vi "CAL-Get MAX SPL (tone, scalar).vi"(0 "Cal Path":path, 7 "Frequency (kHz)":dbl, 11 "error in (no error)":errorcluster) -> (8 "Max SPL":dbl, 15 "error out":errorcluster)   [LabVIEW 2020]
uses:
  PXI DAQ VIs/DAQ Engine VIs/PXI Globals.vi
  Utility VIs/Math VIs/Linear to dB (scalar).vi
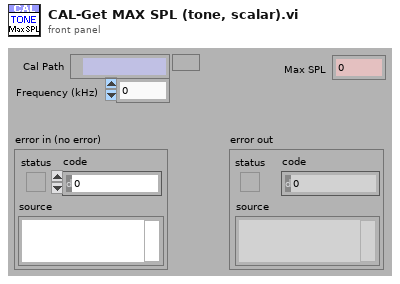
[diagram p1: front panel]
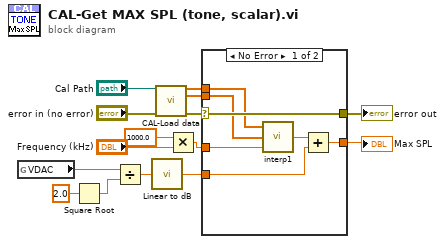
[diagram p0: block diagram]
diagram:
  n1 = global read "PXI Globals.vi" "VDAC"() -> (w5:dbl)
  n2 = Square Root(x=2.0 ("y")) -> (sqrt(x)=w7:dbl)
  n3 = Divide(x=w5, y=w7) -> (x/y=w6:dbl)
  n4 = call-poly "Linear to dB.vi"("Linear"=w6) -> ("dB"=w8:dbl)
  n5 = call "CAL-Load data.vi"("user path"="Cal Path", "error in (no error)"="error in (no error)") -> ("Frequency (Hz)"=w12:dbl[], "Mag"=w1:dbl[], "error out"=w14:errorcluster)  [unwired: 6 in, 5 out]
  n6 = Multiply(x=1000.0, y="Frequency (kHz)") -> (x*y=w4:dbl)
  n7 = case shown="No Error" w14 {
    selector: w14 -> [w22 w23]
    tunnel: [w22 w23] -> w13
    tunnel: w1 -> [w16 _]
    tunnel: w12 -> [w17 _]
    tunnel: w4 -> [w21 _]
    tunnel: [w20 _] -> w10
    tunnel: w8 -> [w18 _]
    frame No Error {
      n8 = call "interp1.vi"("X"=w17, "Y"=w16, "U"=w21) -> ("V"=w19:dbl)  [unwired: 2 in]
      n9 = Add(x=w19, y=w18) -> (x+y=w20:dbl)
    }
    frame Error {
    }
  }
  "error out" <- w13
  "Max SPL" <- w10
